vi "SET_Locked_ActiveLayer.vi"(8 "error in (no error)":errorcluster, 9 "Layers Locked?":bool, 10 "Active Layer":i32, 11 "Icon.lvclass in":refnum<class "Icon.lvclass">) -> (0 "error out":errorcluster, 3 "Icon.lvclass out":refnum<class "Icon.lvclass">)   [LabVIEW 2021, in "Icon.lvclass"]
doc: "Specifies the active User Layer and wheter or not it is locked."
uses:
  Icon.lvclass
  Icon.lvclass/Icon.ctl
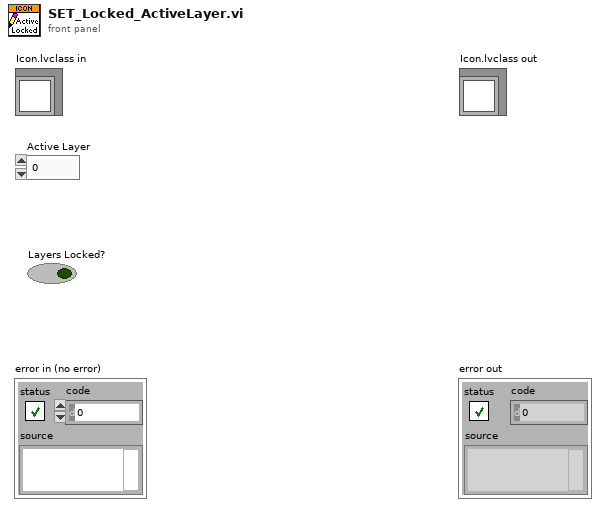
[diagram p1: front panel]
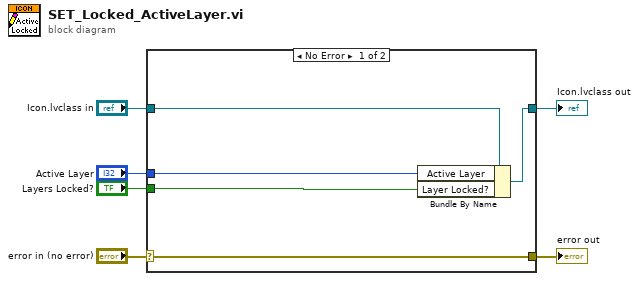
[diagram p0: block diagram]
diagram:
  n1 = case shown="No Error" "error in (no error)" {
    selector: "error in (no error)" -> [w11 w12]
    tunnel: [w11 w12] -> w5
    tunnel: [w9 w13] -> w3
    tunnel: "Icon.lvclass in" -> [w10 w13]
    tunnel: "Active Layer" -> [w8 _]
    tunnel: "Layers Locked?" -> [w7 _]
    frame No Error {
      n2 = Bundle By Name(cluster=w10, "Active Layer"=w8, "Layer Locked?"=w7) -> (w9:refnum<class "Icon.lvclass">)
    }
    frame Error {
    }
  }
  "error out" <- w5
  "Icon.lvclass out" <- w3
